vi "SONAR.vi"() -> ()   [LabVIEW 2020]
uses:
  <vilib>/picture/picture.llb/imagedata.ctl
  <vilib>/MakerHub/LINX/Public/Utilities/Open Serial.vi
  <vilib>/MakerHub/LINX/Public/Sensors/Motion/Servo/Servo Open One Channel.vi
  <vilib>/MakerHub/LINX/Public/Sensors/Motion/Servo/Servo Set Pulse Width One Channel.vi
  <vilib>/MakerHub/LINX/Public/Sensors/Motion/Servo/Servo Close One Channel.vi
  <vilib>/MakerHub/LINX/LMH-LINX.lvlib
  <vilib>/MakerHub/LINX/Public/Sensors/Motion/Servo/Servo.lvlib
  <vilib>/MakerHub/LINX/Public/Sensors/Distance/Ultrasonic/Ultrasonic.lvlib
  <vilib>/ptbypt/NI_PtbyPt.lvlib
panel:
  out "Position":string
  out "Degrees":dbl format="%#_3f"
  out "Distance":dbl caption="CM" format="%#_4f"
  out "2D Picture":picture
  in  "Stop":bool
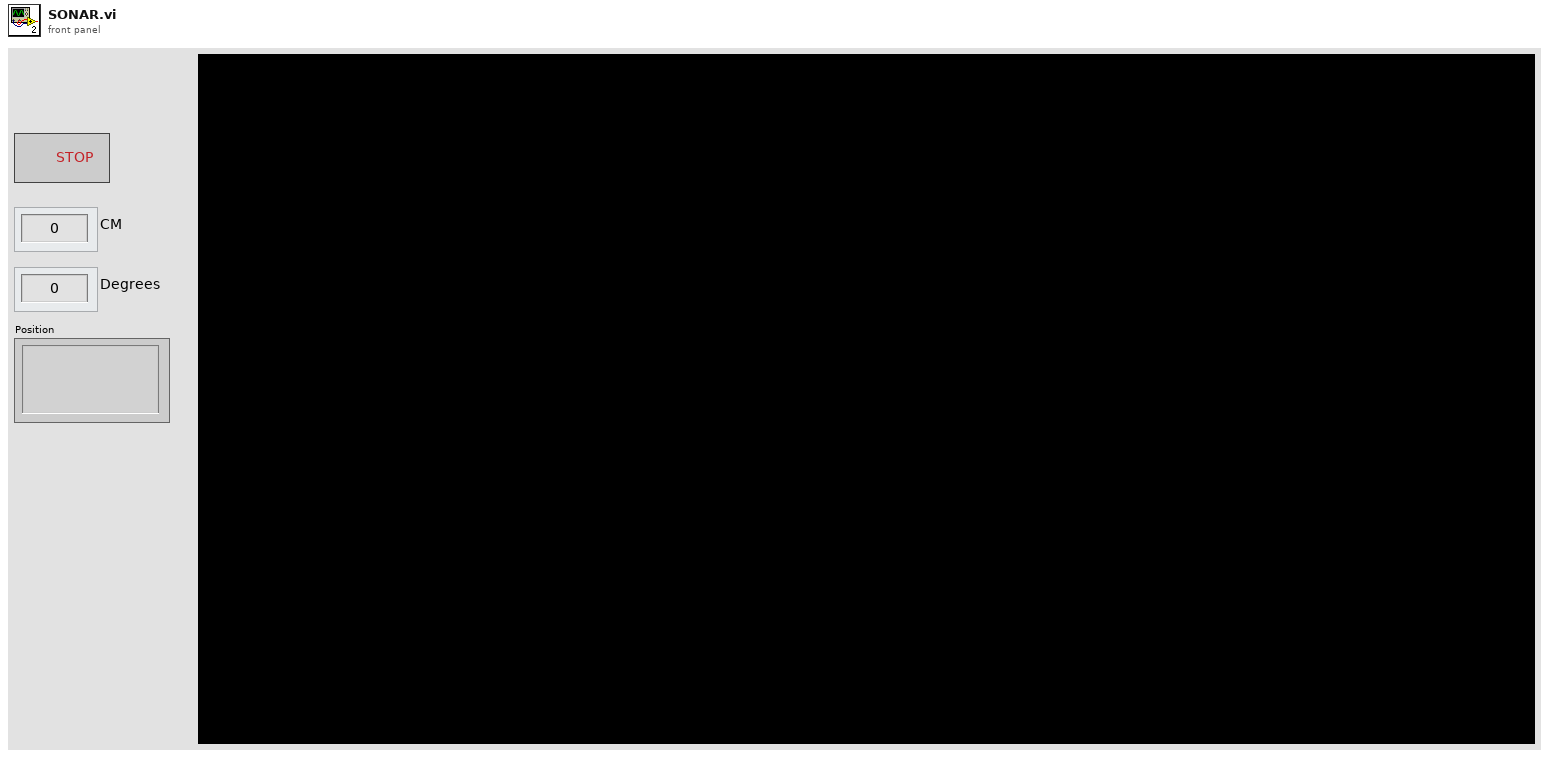
[diagram p1: front panel]
types:
  T1 = typedef "imagedata.ctl" = cluster{"image type":i32, "image depth":i32, "image":u8[], "mask":u8[], "colors":u32[], "Rectangle":cluster{"left":i16, "top":i16, "right":i16, "bottom":i16}}
  T2 = typedef "LMH-LINX.lvlib/LINX Ref.ctl" = cluster{"IO":T3, "Interface":T4, "LINX Device Config":T5}
  T3 = typedef "LMH-LINX.lvlib/Platform.ctl" = enum16{"Remote", "Local"}
  T4 = typedef "LMH-LINX.lvlib/Interface.ctl" = enum16{"Serial", "TCP"}
  T5 = typedef "LMH-LINX.lvlib/Device.lvlib/LINX Device Config.ctl" = cluster{"Interface":T4, "COM Port":refnum<visa-resource-name>, "TCP Configuration":T6, "Device Family":u8, "Device ID":u8, "Device Name":string, "TCP Ref":refnum<k5>, "Channels":T7}
  T6 = typedef "LMH-LINX.lvlib/Device.lvlib/TCP Config.ctl" = cluster{"IP Address":string, "Port":u16}
  T7 = typedef "LMH-LINX.lvlib/Channels.ctl" = cluster{"DI":u8[], "DO":u8[], "AI":u8[], "AO":u8[], "PWM":u8[], "QE":u8[], "UART":u8[], "I2C 2":u8[], "SPI":u8[], "CAN":u8[], "Servo":u8[], "AI Ref (V)":dbl, "AI Resolution (Bits)":u8, "AO Ref (V)":dbl, "AO Resolution (Bits)":u8}
  T8 = cluster{"maximum":dbl, "minimum":dbl, "clip to min":bool, "log?(F)":bool, "grid color":u32, "plot color":u32, "format and precision":cluster{"format":enum8{"Decimal", "Scientific", "Engineering", "Binary", "Octal", "Hex"}, "precision":u8}, "visible section":u16}
  T9 = typedef "LVBoundsTypeDef.ctl" = cluster{"Width":u32, "Height":u32}
  T10 = cluster{"pixel center":cluster{"x":i16, "y":i16}, "scale factors":cluster{"a":dbl, "b":dbl, "log?":bool}, "grid color":u32, "start angle":dbl, "end angle":dbl, "tick length":i16, "pixel radius":i32}
  T11 = cluster{"Distance (cm)":dbl, "Angle (Deg)":dbl}[]
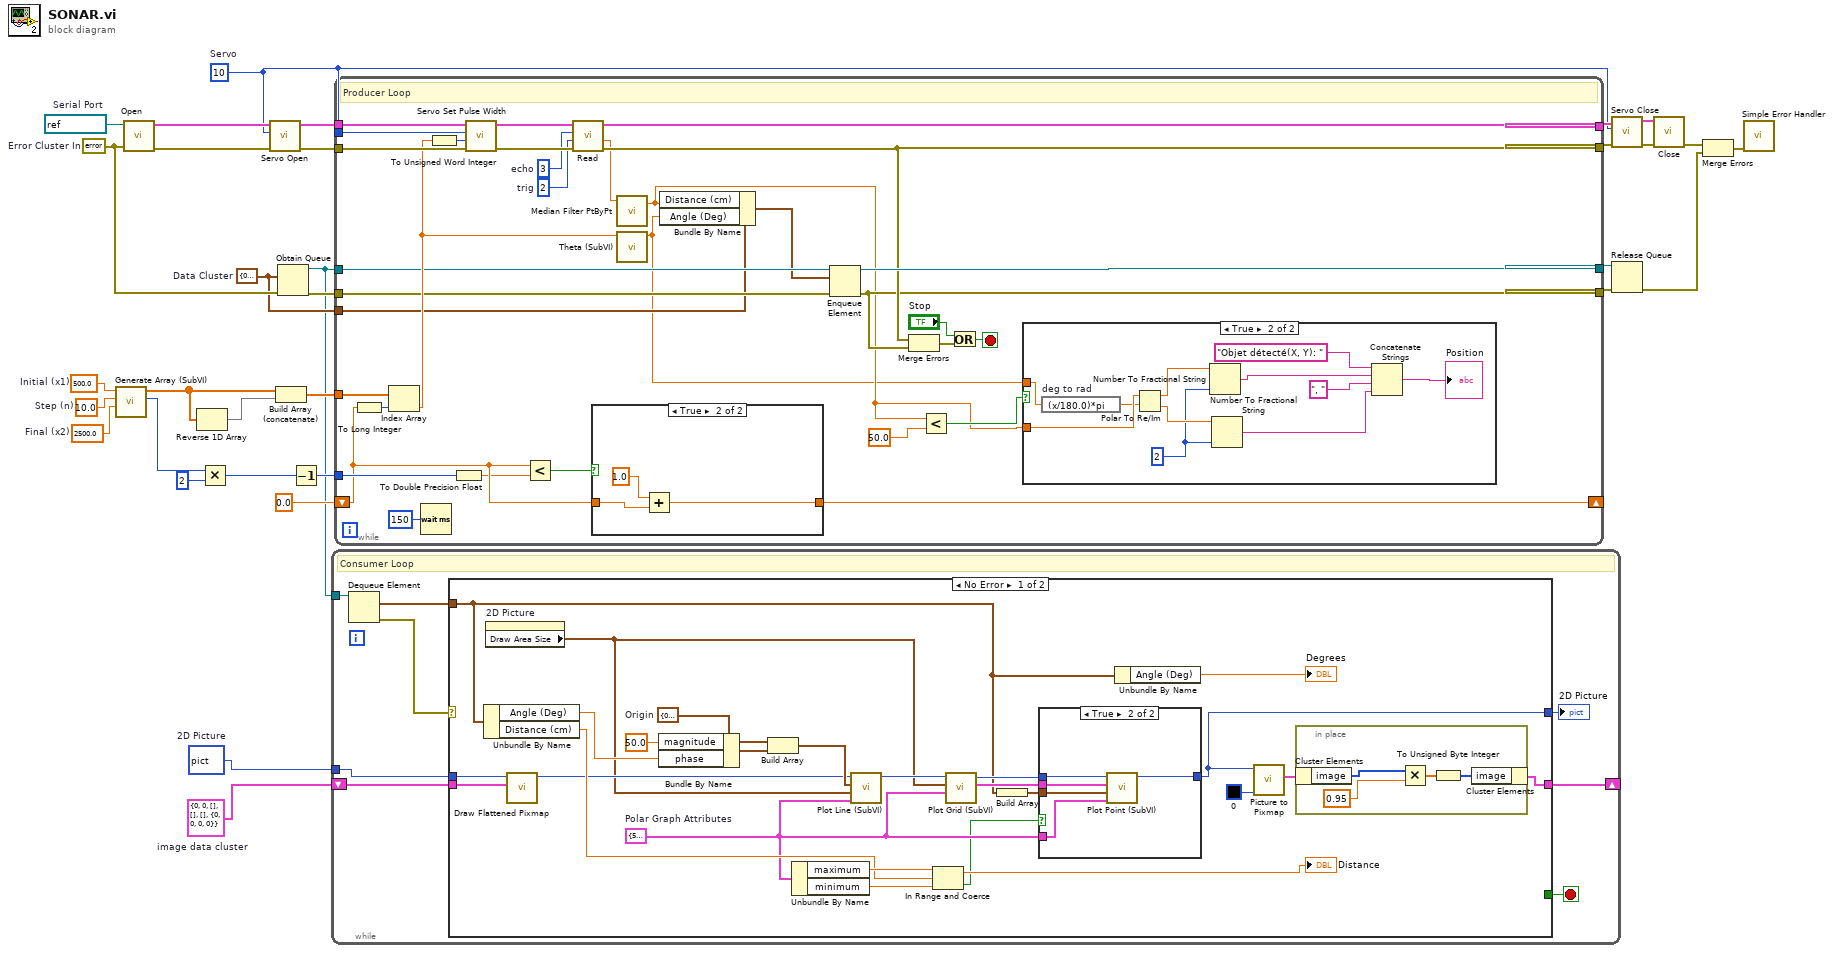
[diagram p0: block diagram]
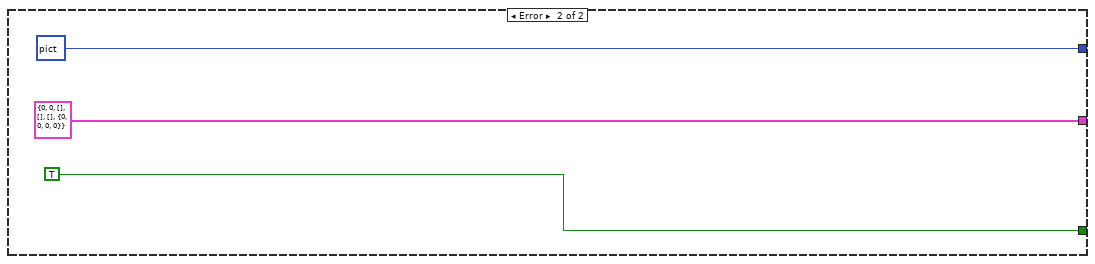
[diagram p3: hidden frame]
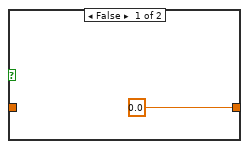
[diagram p5: hidden frame]
diagram:
  w1 = T1 {"image type"=0, "image depth"=0, "image"=[], "mask"=[], "colors"=[], "Rectangle"={"left"=0, "top"=0, "right"=0, "bottom"=0}}  # image data cluster
  w2 = picture data[5B]  # 2D Picture
  w7 = cluster{"Distance (cm)":dbl, "Angle (Deg)":dbl} {"Distance (cm)"=0.0, "Angle (Deg)"=0.0}  # Data Cluster
  w20 = 2500.0  # Final (x2)
  w19 = 10.0  # Step (n)
  w18 = 500.0  # Initial (x1)
  w23 = u8 10  # Servo
  w10 = errorcluster {"status"=FALSE, "code"=0, "source"=""}  # Error Cluster In
  w32 = refnum<visa-resource-name> "COM3"  # Serial Port
  n1 = call "Generate Array (SubVI).vi"("Final"=w20, "Step"=w19, "Initial"=w18) -> ("Array size"=w13:i32, "Array out"=w16:dbl[])  [unwired: 6 in, 1 out]
  n2 = call-poly <vilib>:"Open.vi"("Error In"=w10, "Serial Port"=w32) -> ("Error Out"=w28:errorcluster, "LINX Resource"=w29:T2)  [unwired: 7 in, 1 out]
  n3 = Reverse 1D Array(array=w16) -> (reversed array=w15:dbl[])
  n4 = Multiply(x=w13, y=2) -> (x*y=w14:i32)
  n5 = call-poly <vilib>:"Servo Open.vi"("Error In"=w28, "Servo Channel"=w23, "LINX Resource"=w29) -> ("Error Out"=w26:errorcluster, "LINX Resource"=w27:T2)  [unwired: 7 in]
  n6 = Build Array (concatenate)(w16, w15) -> (w17:dbl[])
  n7 = Obtain Queue(element data type=w7, error in (no error)=w10) -> (queue out=w3:refnum<queue>, error out=w11:errorcluster)  [unwired: 3 in, 1 out]
  n8 = Decrement(x=w14) -> (x-1=w21:i32)
  n9 = while {
    tunnel: w3 -> [w33]
    tunnel: w2 -> [w37]
    shift-right: [w34] -> _
    shift-left: w1 -> [w36]
    stop <- w38 stop-if-true
    # "Consumer Loop"
    n10 = Dequeue Element(queue=w33) -> (element=w39:cluster{"Distance (cm)":dbl, "Angle (Deg)":dbl}, error out=w40:errorcluster)  [unwired: 2 in, 2 out]
    n11 = case shown="No Error" w40 {
      tunnel: w39 -> [w49 _]
      tunnel: [_ TRUE] -> w38
      tunnel: w37 -> [w65 _]
      tunnel: w36 -> [w64 _]
      tunnel: [w60 picture data[5B] ("new picture")] -> w35
      tunnel: [w63 T1 {"image type"=0, "image depth"=0, "image"=[], "mask"=[], "colors"=[], "Rectangle"={"left"=0, "top"=0, "right"=0, "bottom"=0}} ("image data")] -> w34
      frame No Error {
        w47 = T8 {"maximum"=50.0, "minimum"=0.0, "clip to min"=TRUE, "log?(F)"=FALSE, "grid color"=9868950, "plot color"=65280, "format and precision"={"format"=enum."Decimal", "precision"=0}, "visible section"=4}  # Polar Graph Attributes
        w43 = cluster{"magnitude":dbl, "phase":dbl} {"magnitude"=0.0, "phase"=0.0}  # Origin
        n12 = Unbundle By Name(w49) -> ("Angle (Deg)"=w53:dbl, "Distance (cm)"=w54:dbl)
        n13 = property on="2D Picture" class="Pict"() -> ("Draw Area Size"=w51:T9)  [unwired: 2 in, 2 out]
        n14 = call <vilib>:"Draw Flattened Pixmap.vi"("image data"=w64, "picture"=w65) -> ("new picture"=w52:picture)  [unwired: 7 in]
        n15 = Bundle By Name(cluster=w43, "magnitude"=50.0, "phase"=w53) -> (w42:cluster{"magnitude":dbl, "phase":dbl})
        n16 = Build Array(w43, w42) -> (w61:cluster{"magnitude":dbl, "phase":dbl}[])
        n17 = Unbundle By Name(w47) -> ("maximum"=w56:dbl, "minimum"=w55:dbl)
        n18 = call "Plot Line (SubVI).vi"("Polar Graph Attributes"=w47, "Draw Area Size"=w51, "Polar Array"=w61, "new picture in"=w52) -> ("new picture out"=w62:picture)  [unwired: 7 in]
        n19 = In Range and Coerce(upper limit=w56, x=w54, lower limit=w55) -> (coerced(x)=→"Distance":dbl, In Range?=w41:bool)
        n20 = call "Plot Grid (SubVI).vi"("Polar Graph Attributes"=w47, "Draw Area Size"=w51, "new picture in"=w62) -> ("grid measurements"=w58:T10, "new picture out"=w59:picture)  [unwired: 7 in]
        n21 = Build Array(w49) -> (w50:T11)
        n22 = case shown="True" w41 {
          tunnel: w50 -> [_ w71]
          tunnel: [w70 w75] -> w60
          tunnel: w59 -> [w70 w73]
          tunnel: w58 -> [_ w72]
          tunnel: w47 -> [_ w74]
          frame False {
            # "Nothing Detected"
          }
          frame True {
            # "Plot and scale object to 2D picture"
            n23 = call "Plot Point (SubVI).vi"("Polar Graph Attributes"=w74, "Array"=w71, "grid measurements"=w72, "new picture in"=w73) -> ("new picture"=w75:picture)  [unwired: 7 in]
          }
        }
        n24 = Unbundle By Name(w49) -> ("Angle (Deg)"=→"Degrees":dbl)
        n25 = call <vilib>:"Picture to Pixmap.vi"("Background Color"=u32 0, "picture"=w60) -> ("image data"=w46:T1)  [unwired: 8 in, 1 out]
        n26 = in-place {
          # "Ghosting Effect"
          n27 = in-place-cluster #1(w46) -> ("image"=w69:u8[])
          n28 = Multiply(x=w69, y=0.95) -> (x*y=w67:dbl[])
          n29 = To Unsigned Byte Integer(number=w67) -> (unsigned 8bit integer=w66:u8[])
          n30 = in-place-cluster #1("image"=w66) -> (w63:T1)
        }
      }
      frame Error {
      }
    }
    "2D Picture" <- w35
  }
  n31 = while {
    tunnel: [w102] -> w31
    tunnel: [w90] -> w30
    tunnel: w27 -> [w104]
    tunnel: w26 -> [w105]
    tunnel: w23 -> [w110]
    tunnel: w17 -> [w109]
    shift-right: [w98] -> _
    shift-left: 0.0 -> [w107]
    tunnel: w21 -> [w108]
    tunnel: w7 -> [w93]
    tunnel: w11 -> [w96]
    tunnel: [w89] -> w8
    tunnel: w3 -> [w95]
    tunnel: [w94] -> w9
    stop <- w111 stop-if-true
    w99 = u8 2  # trig
    w100 = u8 3  # echo
    # "Producer Loop"
    n32 = To Long Integer(number=w107) -> (32bit integer=w85:i32)
    n33 = Index Array "Index Array"(array=w109, index=w85) -> (element=w97:dbl)
    n34 = Wait (ms)(milliseconds to wait=u32 150 ("Slide")) -> ()  [unwired: 1 out]
    n35 = To Unsigned Word Integer(number=w97) -> (unsigned 16bit integer=w86:u16)
    n36 = To Double Precision Float(number=w108) -> (double precision float=w84:dbl)
    n37 = call-poly <vilib>:"Servo Set Pulse Width.vi"("Error In"=w105, "Pulse Width (uS)"=w86, "Servo Channel"=w110, "LINX Resource"=w104) -> ("Error Out"=w101:errorcluster, "LINX Resource"=w103:T2)  [unwired: 6 in]
    n38 = Less?(x=w107, y=w84) -> (x < y?=w106:bool)
    n39 = call <vilib>:"Read.vi"("Error In"=w101, "DO Channel"=w99, "DI Channel"=w100, "LINX Resource"=w103) -> ("Error Out"=w90:errorcluster, "Centimeters"=w83:dbl, "LINX Resource"=w102:T2)  [unwired: 4 in, 1 out]
    n40 = case shown="True" w106 {
      tunnel: [0.0 w126] -> w98
      tunnel: w107 -> [_ w125]
      frame False {
        # "Reset to 0 IF counter greater than array size"
      }
      frame True {
        # "Increment Counter IF less than Array Size"
        n41 = Add(x=1.0, y=w125) -> (x+y=w126:dbl)
      }
    }
    n42 = call <vilib>:"Median Filter PtByPt.vi"("x"=w83) -> ("Filtered x"=w80:dbl)  [unwired: 3 in, 1 out]
    n43 = call "Theta (SubVI).vi"("PWM"=w97) -> ("Theta"=w79:dbl)  [unwired: 9 in, 1 out]
    n44 = Bundle By Name(cluster=w93, "Distance (cm)"=w80, "Angle (Deg)"=w79) -> (w92:cluster{"Distance (cm)":dbl, "Angle (Deg)":dbl})
    n45 = Enqueue Element(queue=w95, element=w92, error in (no error)=w96) -> (queue out=w94:refnum<queue>, error out=w89:errorcluster)  [unwired: 1 in, 1 out]
    n46 = Merge Errors(w90, w89) -> (w88:errorcluster)
    n47 = Less?(x=w80, y=50.0) -> (x < y?=w81:bool)
    n48 = Or(x="Stop", y=w88) -> (x .or. y?=w111:bool)
    n49 = case shown="True" w81 {
      tunnel: w79 -> [_ w112]
      tunnel: w80 -> [_ w119]
      frame False {
      }
      frame True {
        w114 = i16 2 ("precision (6)")
        n50 = expression code="(x/180.0)*pi" "deg to rad"(w112) -> (w113:dbl)
        n51 = Polar To Re/Im(2:w113, 3:w119) -> (0:w118:dbl, 1:w117:dbl)
        n52 = Number To Fractional String(number=w117, precision (6)=w114) -> (F-format string=w116:string)  [unwired: 2 in]
        n53 = Number To Fractional String(number=w118, precision (6)=w114) -> (F-format string=w115:string)  [unwired: 2 in]
        n54 = Concatenate Strings("Objet détecté(X, Y): " ("string"), w116, ", " ("string"), w115) -> (→"Position":string)
      }
    }
  }
  n55 = call-poly <vilib>:"Servo Close.vi"("Error In"=w30, "Servo Channel"=w23, "LINX Resource"=w31) -> ("Error Out"=w25:errorcluster, "LINX Resource"=w24:T2)  [unwired: 7 in]
  n56 = Release Queue(queue=w9, error in (no error)=w8) -> (error out=w4:errorcluster)  [unwired: 1 in, 2 out]
  n57 = call <vilib>:"Close.vi"("Error In"=w25, "LINX Resource"=w24) -> ("Error Out"=w6:errorcluster)  [unwired: 9 in]
  n58 = Merge Errors(w6, w4) -> (w5:errorcluster)
  n59 = call <vilib>:"Simple Error Handler.vi"("error in (no error)"=w5) -> ()  [unwired: 4 in, 5 out]
